vi "GetImageandProduceSplitDimensions.vi"(11 "Row/Column [].Length":i32) -> (0 "Draw Image Size X":i32, 1 "Image Subset Y Length":i32, 2 "Selected Image":T1, 3 "Image Subset X Length":i32, 4 "Draw Image Size Y":i32)   [LabVIEW 2020]
uses:
  <vilib>/picture/picture.llb/imagedata.ctl
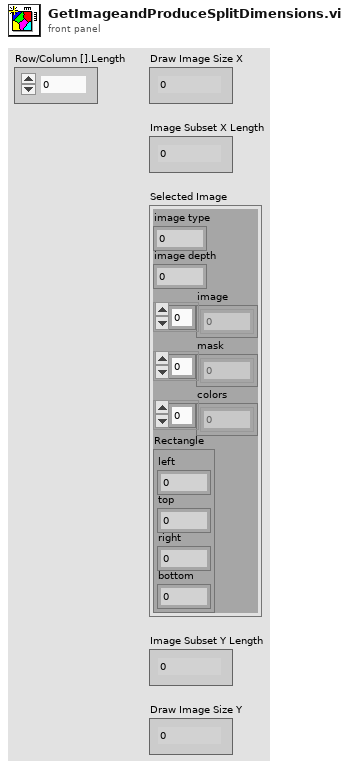
[diagram p1: front panel]
types:
  T1 = typedef "imagedata.ctl" = cluster{"image type":i32, "image depth":i32, "image":u8[], "mask":u8[], "colors":u32[], "Rectangle":cluster{"left":i16, "top":i16, "right":i16, "bottom":i16}}
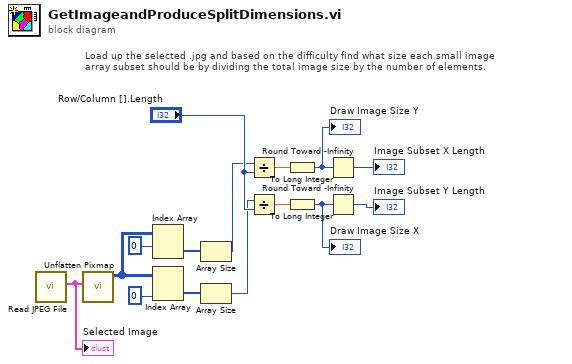
[diagram p0: block diagram]
diagram:
  # "Load up the selected .jpg and based on the difficulty find what size each small image \narray subset should be by dividing the total image size by the number of elements."
  n1 = call <vilib>:"Read JPEG File.vi"() -> ("image data"=w12:T1)  [unwired: 9 in, 2 out]
  "Selected Image" <- w12
  n2 = call <vilib>:"Unflatten Pixmap.vi"("image data"=w12) -> ("24-bit pixmap"=w5:u32[][])  [unwired: 4 in, 6 out]
  n3 = Index Array(array=w5, index (row)=0) -> (element=w8:u32[])  [unwired: 1 in]
  n4 = Index Array(array=w5, index (col)=0 ("disabled index (col)")) -> (element=w9:u32[])  [unwired: 1 in]
  n5 = Array Size(array=w8) -> (size(s)=w10:i32)
  n6 = Array Size(array=w9) -> (size(s)=w11:i32)
  n7 = Divide(x=w10, y="Row/Column [].Length") -> (x/y=w4:dbl)
  n8 = Divide(x=w11, y="Row/Column [].Length") -> (x/y=w2:dbl)
  n9 = To Long Integer(number=w4) -> (32bit integer=w3:i32)
  "Draw Image Size Y" <- w3
  n10 = To Long Integer(number=w2) -> (32bit integer=w1:i32)
  "Draw Image Size X" <- w1
  n11 = Round Toward -Infinity(1:w3) -> (0:→"Image Subset X Length":i32)
  n12 = Round Toward -Infinity(1:w1) -> (0:→"Image Subset Y Length":i32)
